vi "Launch Job.vi"(8 "error in (no error)":errorcluster, 9 "Reply Queue":refnum<queue>, 10 "Job.lvclass":refnum<class "Job.lvclass">, 11 "CI Mediator in":refnum<class "CI Mediator.lvclass">) -> (0 "error out":errorcluster, 3 "CI Mediator out":refnum<class "CI Mediator.lvclass">)   [LabVIEW 2014, in "CI Mediator.lvlib" / "CI Mediator.lvclass"]
uses:
  CI Mediator.lvclass
  Classes/Job/Job.lvclass
  Controls/Job Results - STYP.ctl
  Jobber Proxy/Jobber Proxy/Jobber Proxy.lvclass
  Jobber Proxy/Jobber Proxy/Jobber Proxy.lvclass/Jobber Proxy.ctl
  Classes/Job/Job.lvclass/Job.ctl
  CI Mediator.lvclass/CI Mediator.ctl
  Classes/Executor/Executor.lvclass
  Classes/Log File/Log File.lvclass
  <vilib>/ActorFramework/Actor/Actor.lvclass
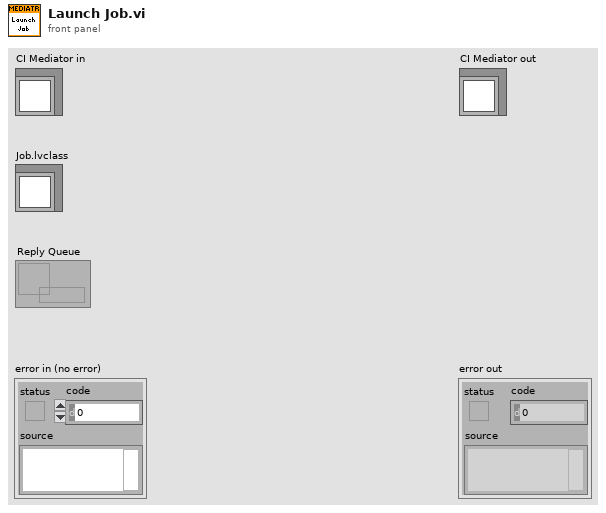
[diagram p1: front panel]
types:
  T1 = typedef "Executor Status - STYP.ctl" = cluster{"Executor Name":string, "Status":bool}
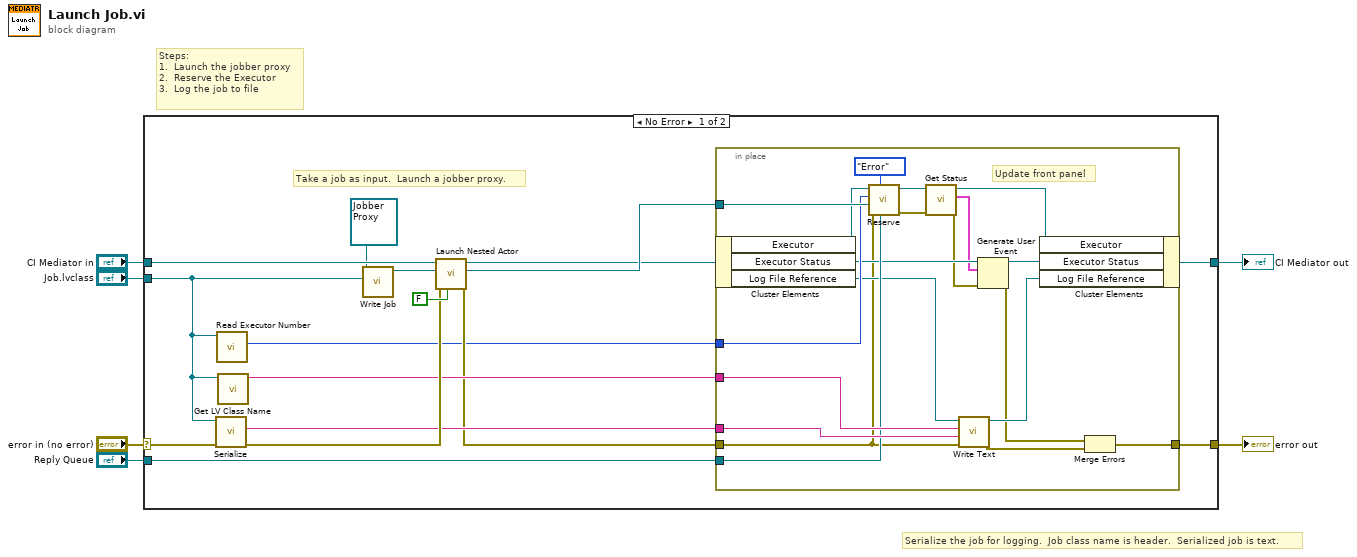
[diagram p0: block diagram]
diagram:
  # "Steps:\n1.  Launch the jobber proxy\n2.  Reserve the Executor\n3.  Log the job to file"
  # "Serialize the job for logging.  Job class name is header.  Serialized job is text."
  n1 = case shown="No Error" "error in (no error)" {
    selector: "error in (no error)" -> [w21 w44]
    tunnel: [w22 w44] -> w5
    tunnel: [w12 w43] -> w3
    tunnel: "CI Mediator in" -> [w11 w43]
    tunnel: "Job.lvclass" -> [w7 _]
    tunnel: "Reply Queue" -> [w10 _]
    frame No Error {
      # "Take a job as input.  Launch a jobber proxy."
      n2 = call-dynamic "Serialize.vi"("error in (no error)"=w21, "Job in"=w7) -> ("error out"=w18:errorcluster, "Text"=w17:string)  [unwired: 8 in]
      n3 = call "Read Executor Number.vi"("Job in"=w7) -> ("Executor Number"=w14:i32)  [unwired: 8 in, 2 out]
      n4 = call <vilib>:"Get LV Class Name.vi"("object"=w7) -> ("class name"=w16:string)  [unwired: 9 in, 1 out]
      n5 = call "Write Job.vi"("Job.lvclass"=w7, "Jobber Proxy in"=refnum<class "Jobber Proxy.lvclass"> refnum ("Jobber Proxy.lvlib:Jobber Proxy.lvclass")) -> ("Jobber Proxy out"=w9:refnum<class "Jobber Proxy.lvclass">)  [unwired: 9 in]
      n6 = call <vilib>:"Launch Nested Actor.vi"("Open Actor Core front panel? (F)"=FALSE, "error in (no error)"=w18, "Nested Actor"=w9, "Caller Actor in"=w11) -> ("error out"=w15:errorcluster, "Nested Actor's Enqueuer"=w19:refnum<class "Message Enqueuer.lvclass">, "Caller Actor out"=w13:refnum<class "CI Mediator.lvclass">)  [unwired: 5 in]
      n7 = in-place {
        in-place-border: [w25] -> w22
        in-place-border: w19 -> [w40]
        in-place-border: w17 -> [w39]
        in-place-border: w16 -> [w38]
        in-place-border: w15 -> [w23]
        in-place-border: w14 -> [w37]
        in-place-border: w10 -> [w35]
        # "Update front panel"
        n8 = in-place-cluster #1(w13) -> ("Executor"=w36:refnum<class "Executor.lvclass">, "Executor Status"=w31:refnum<user-event>, "Log File Reference"=w28:refnum<data-value>)
        n9 = call "Reserve.vi"("Reply Queue"=w35, "Overbook Reserve Action"=enum16{"Error", "Override"}."Error", "error in (no error)"=w23, "Actor Enquerer"=w40, "Executor Number"=w37, "Executor"=w36) -> ("error out"=w32:errorcluster, "Executor"=w34:refnum<class "Executor.lvclass">)  [unwired: 4 in]
        n10 = call "Get Status.vi"("error in (no error)"=w32, "Executor Reference"=w34) -> ("error out"=w26:errorcluster, "Status[]"=w29:T1[], "Executor Reference"=w33:refnum<class "Executor.lvclass">)  [unwired: 6 in, 1 out]
        n11 = call "Write Text.vi"("error in (no error)"=w23, "Text"=w39, "Header"=w38, "Log File Ref"=w28) -> ("error out"=w42:errorcluster, "Log File Ref"=w27:refnum<data-value>)  [unwired: 6 in]
        n12 = Generate User Event(user event=w31, event data cluster=w29, error in=w26) -> (user event out=w30:refnum<user-event>, error out=w24:errorcluster)  [unwired: 1 in]
        n13 = in-place-cluster #1("Executor"=w33, "Executor Status"=w30, "Log File Reference"=w27) -> (w12:refnum<class "CI Mediator.lvclass">)
        n14 = Merge Errors(w24, w42) -> (w25:errorcluster)
      }
    }
    frame Error {
    }
  }
  "error out" <- w5
  "CI Mediator out" <- w3
